vi "CAN Send.vi"(8 "error in (no error)":errorcluster, 9 "data":u8[](array[numeric]), 10 "messageID":u32 format="%.0x") -> (0 "error out":errorcluster)   [LabVIEW 2009, in "CAN.lvlib"]
uses:
  CAN.lvlib
  Serial.lvlib
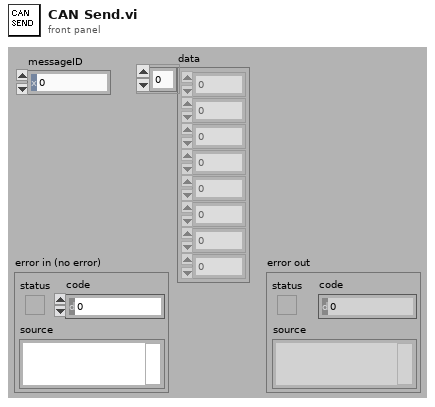
[diagram p1: front panel]
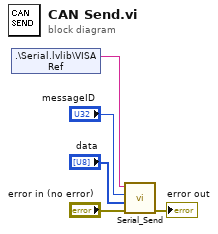
[diagram p0: block diagram]
diagram:
  n1 = shared-variable ".\\Serial.lvlib\\VISA Ref"() -> (w5:string)  [unwired: 1 in, 1 out]
  n2 = call "Serial_Send.vi"("error in"="error in (no error)", "data"="data", "messageID"="messageID", "VISA resource name"=w5) -> ("error out"=→"error out":errorcluster)  [unwired: 6 in, 1 out]
